vi "Go to Voltage.vi"(8 "error in":errorcluster, 10 "Set Voltage":dbl min=0.0 max=700.0, 11 "VISA Resource Name":refnum<visa-resource-name>) -> (0 "error out":errorcluster, 2 "Actual Voltage":dbl, 3 "VISA resource name out":refnum<visa-resource-name>)   [LabVIEW 2017]
panel:
  in  "Output Terminal":tag="/Dev1/PFI4"
  in  "Counter":tag="Dev1/ctr0"
  in  "Stop":bool
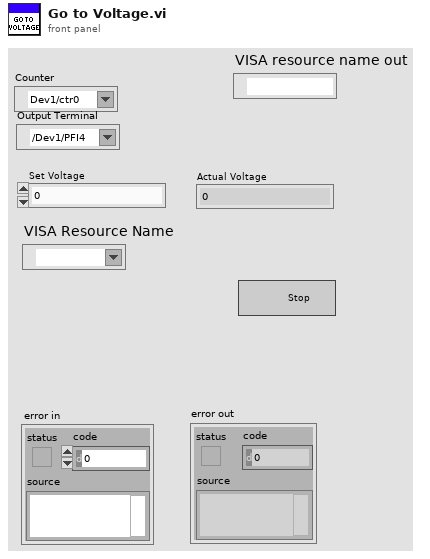
[diagram p1: front panel]
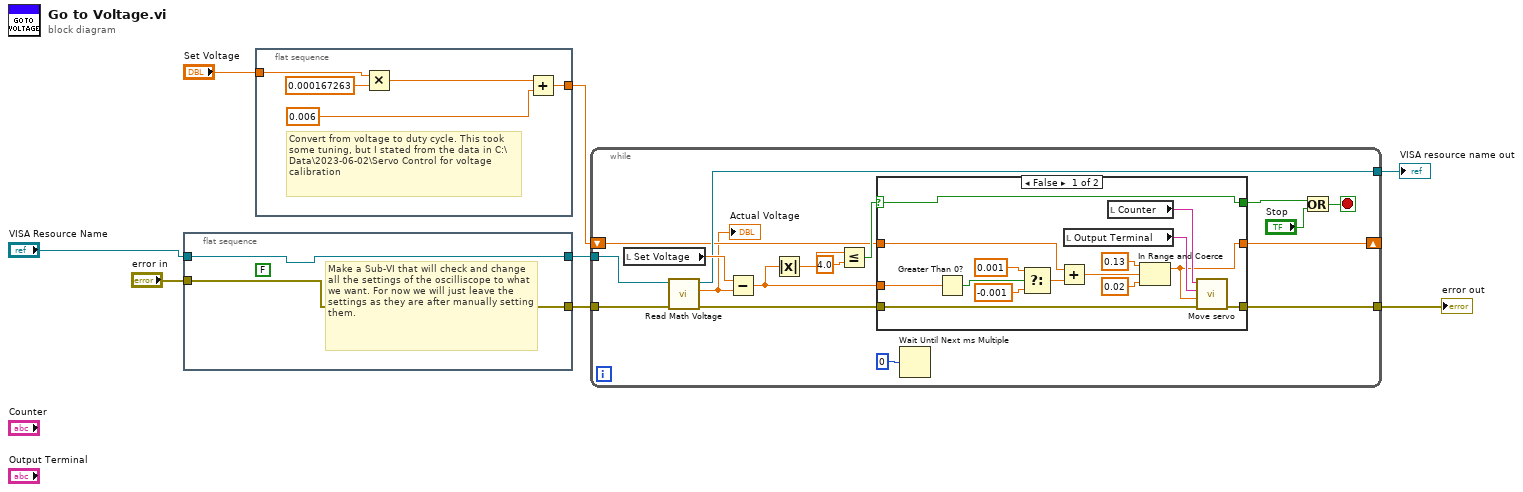
[diagram p0: block diagram]
diagram:
  n1 = flat-sequence {
    tunnel: [w9] -> w8
    tunnel: [w10] -> w7
    tunnel: "error in" -> [w9]
    tunnel: "VISA Resource Name" -> [w10]
    frame #0 {
      (unwired) FALSE ("Reset? (T: Yes)")
      # "Make a Sub-VI that will check and change all the settings of the oscilliscope to what we want. For now we will just leave the settings as they are after manually setting them."
    }
  }
  n2 = flat-sequence {
    tunnel: "Set Voltage" -> [w15]
    tunnel: [w11] -> w3
    frame #0 {
      # "Convert from voltage to duty cycle. This took some tuning, but I stated from the data in C:\\Data\\2023-06-02\\Servo Control for voltage calibration"
      n3 = Multiply(x=w15, y=0.000167263) -> (x*y=w14:dbl)
      n4 = Add(x=w14, y=0.006) -> (x+y=w11:dbl)
    }
  }
  n5 = while {
    tunnel: w8 -> [w28]
    tunnel: w7 -> [w27]
    tunnel: [w26] -> w4
    tunnel: [w23] -> w1
    shift-right: [w19] -> _
    shift-left: w3 -> [w18]
    stop <- w22 stop-if-true
    n6 = local read "Set Voltage"() -> (w29:dbl)
    n7 = call "Read Math Voltage.vi"("error in (no error)"=w28, "VISA resource name"=w27) -> ("error out"=w24:errorcluster, "amplitude"=w16:dbl, "VISA resource name out"=w26:refnum<visa-resource-name>)  [unwired: 7 in]
    "Actual Voltage" <- w16
    n8 = Subtract(x=w29, y=w16) -> (x-y=w17:dbl)
    n9 = Absolute Value(x=w17) -> (abs(x)=w31:dbl)
    n10 = Less Or Equal?(x=w31, y=4.0) -> (x <= y?=w25:bool)
    n11 = case shown="False" w25 {
      selector: w25 -> [w43 w49]
      tunnel: w24 -> [w45 w50]
      tunnel: [w44 w50] -> w23
      tunnel: [w43 w49] -> w20
      tunnel: [w35 w48] -> w19
      tunnel: w18 -> [w37 w48]
      tunnel: w17 -> [w42 _]
      frame False {
        n12 = Greater Than 0?(x=w42) -> (x > 0?=w41:bool)
        n13 = Select(t=0.001, s=w41, f=-0.001) -> (s? t:f=w38:dbl)
        n14 = Add(x=w37, y=w38) -> (x+y=w36:dbl)
        n15 = local read "Output Terminal"() -> (w47:tag)
        n16 = local read "Counter"() -> (w46:tag)
        n17 = In Range and Coerce(upper limit=0.13, x=w36, lower limit=0.02) -> (coerced(x)=w35:dbl)  [unwired: 1 out]
        n18 = call "Move servo.vi"("error in"=w45, "Duty Cycle"=w35, "Output Terminal"=w47, "Counter"=w46) -> ("error out"=w44:errorcluster)  [unwired: 6 in, 1 out]
      }
      frame True {
      }
    }
    n19 = Wait Until Next ms Multiple(millisecond multiple=u32 0) -> ()  [unwired: 1 out]
    n20 = Or(x=w20, y="Stop") -> (x .or. y?=w22:bool)
  }
  "error out" <- w1
  "VISA resource name out" <- w4
